vi "Weather Station UI.vi"(7 "stop":bool, 9 "Limite inférieure":dbl=10.0 min=0.0 max=50.0, 10 "Limite supérieure":dbl=30.0 min=0.0 max=50.0) -> (1 "Mise en garde":string, 2 "Historique de la température":dbl(graph))   [LabVIEW 2009]
doc: "Ceci est le VI principal du Projet Station météo. Il comporte l'interface utilisateur d'un système de mise en garde concernant la température. La température est mesurée toutes les demi-secondes ; les données sont enregistrées lorsqu'une mise en garde survient.\n\nEntrées utilisateur : Limite supérieure de température, Limite inférieure de température, Unités de température.\nSorties : Température actuelle, État de mise en garde."
uses:
  Supporting Files/Weather Station States.ctl
panel:
  in  "Limite supérieure du vent":dbl(slide)=50.0 scale=0.0..100.0
  out "Historique de la vitesse du vent":dbl(graph)
  in  "Données météo":dynamicdata(graph)
  # "Celsius"
  # "Gamme de température (C)"
  # "Canicule"
  # "Gel"
  # "km/h"
  # "Vitesse maximale du vent sans danger (km/h)"
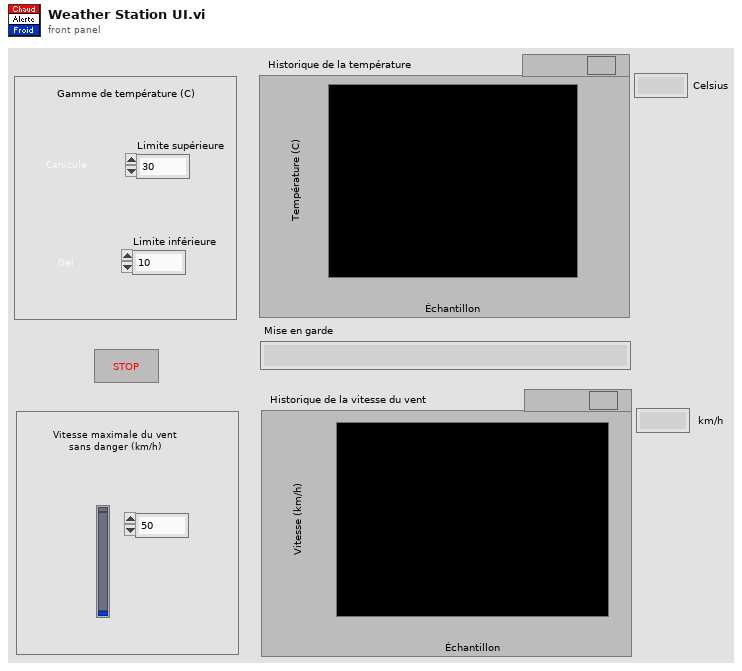
[diagram p1: front panel]
types:
  T1 = cluster{"Température":dbl, "Limite supérieure de T":dbl, "Limite inférieure de T":dbl, "Vitesse du vent":dbl, "Limite supérieure du vent":dbl, "Mise en garde":string, "Temps":dbl}
  T2 = typedef "Weather Station States.ctl" = enum16{"Analyse", "Traiter l'IU", "Définir  la mise en garde", "Enregistrement des  données", "Arrêter"}
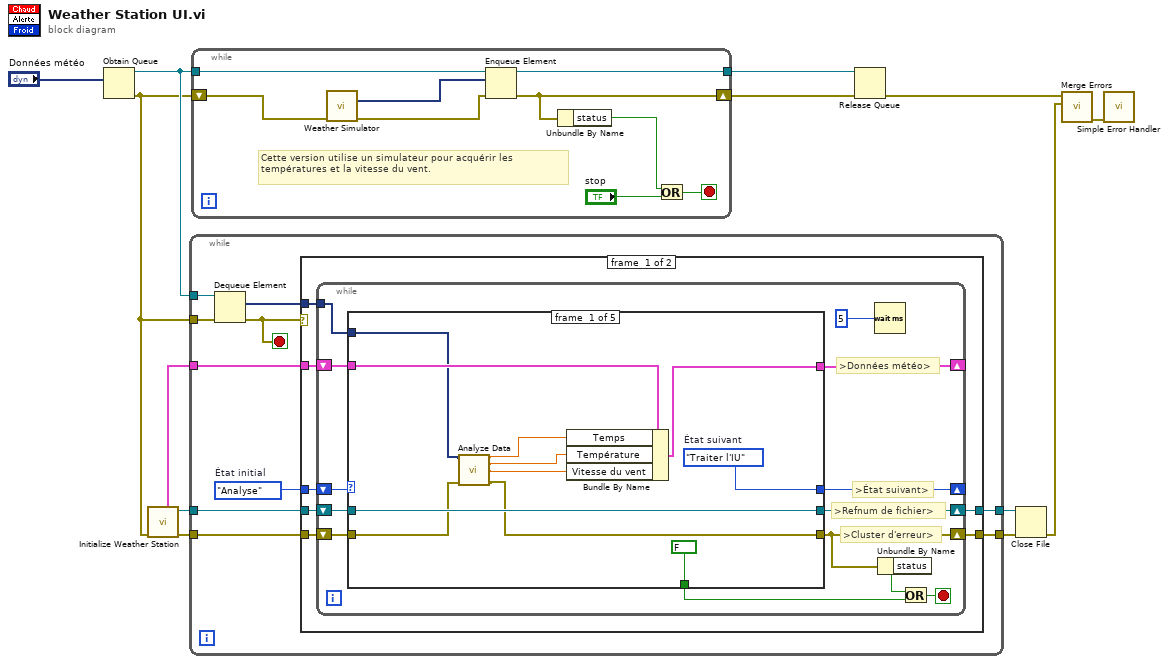
[diagram p0: block diagram]
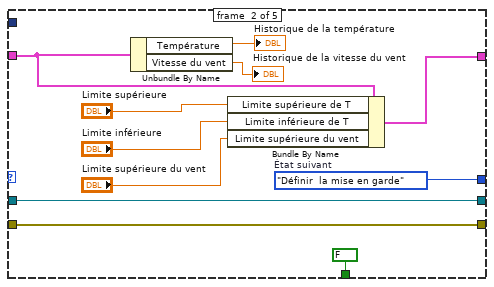
[diagram p2: hidden frame]
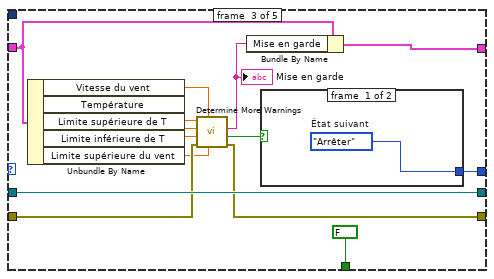
[diagram p3: hidden frame]
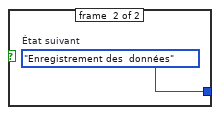
[diagram p4: hidden frame]
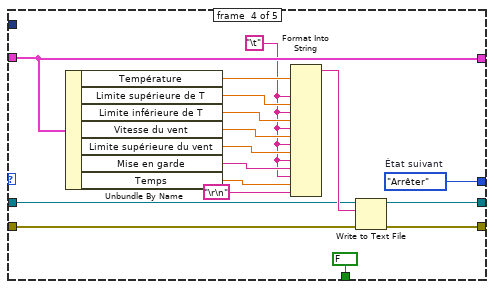
[diagram p5: hidden frame]
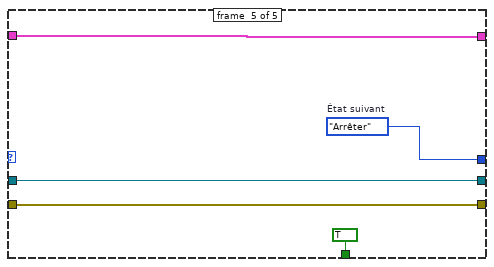
[diagram p6: hidden frame]
diagram:
  n1 = Obtain Queue ("Obtenir une file d'attente")(element data type="Données météo") -> (queue out=w5:refnum<queue>, error out=w1:errorcluster)  [unwired: 4 in, 1 out]
  n2 = call "Initialize Weather Station.vi"("entrée d'erreur (pas d'erreur)"=w1) -> ("sortie d'erreur"=w10:errorcluster, "refnum de fichier"=w11:refnum<file>, "Données météo"=w9:T1)  [unwired: 8 in]
  n3 = while "Boucle While" {
    tunnel: [w23] -> w13
    tunnel: [w22] -> w12
    tunnel: w11 -> [w21]
    tunnel: w10 -> [w20]
    tunnel: w9 -> [w19]
    tunnel: w5 -> [w18]
    tunnel: w1 -> [w17]
    stop <- w16 stop-if-true
    w14 = Weather_Station_States."Analyse"  # État initial
    n4 = Dequeue Element ("Supprimer le premier élément d'une file d'attente")(queue=w18, error in (no error)=w17) -> (element=w15:dynamicdata, error out=w16:errorcluster)  [unwired: 1 in, 2 out]
    n5 = case "Structure Condition" shown="Pas d'erreur" w16 {
      tunnel: w14 -> [w30 _]
      tunnel: [w29 w104] -> w23
      tunnel: [w28 w105] -> w22
      tunnel: w21 -> [w27 w105]
      tunnel: w20 -> [w26 w104]
      tunnel: w19 -> [w25 _]
      tunnel: w15 -> [w24 _]
      frame #0 {
        n6 = while {
          shift-right: [w42] -> _
          shift-left: w30 -> [w43]
          shift-right: [w39] -> w29
          shift-left: w26 -> [w41]
          shift-right: [w32] -> _
          shift-left: w25 -> [w36]
          shift-right: [w37] -> w28
          shift-left: w27 -> [w35]
          tunnel: w24 -> [w31]
          stop <- w40 stop-if-true
          # ">Cluster d'erreur>"
          # ">Données météo>"
          # ">Refnum de fichier>"
          # ">État suivant>"
          n7 = case shown="\"Analyse\"" w43 {
            tunnel: [w54 w59 w77 w98 w99] -> w42
            tunnel: [w47 w60 w70 w96 w101] -> w39
            tunnel: w41 -> [w48 w60 w71 w97 w101]
            tunnel: [w53 w61 w79 w95 w102] -> w37
            tunnel: [w50 w63 w72 w87 w103] -> w32
            tunnel: w36 -> [w51 w55 w73 w87 w103]
            tunnel: w35 -> [w53 w61 w79 w93 w102]
            tunnel: [FALSE ("stop") FALSE ("stop") FALSE ("stop") FALSE ("stop") TRUE ("stop")] -> w34
            tunnel: w31 -> [w49 _ _ _ _]
            frame #0 {
              w54 = Weather_Station_States."Traiter l'IU"  # État suivant
              n8 = call "Analyze Data.vi"("Données météo"=w49, "entrée d'erreur"=w48) -> ("Temps"=w44:dbl, "Température"=w45:dbl, "Vitesse du vent"=w46:dbl, "sortie d'erreur"=w47:errorcluster)  [unwired: 10 in]
              n9 = Bundle By Name(cluster=w51, "Temps"=w44, "Température"=w45, "Vitesse du vent"=w46) -> (w50:T1)
            }
            frame #1 {
              w59 = Weather_Station_States."Définir  la mise en garde"  # État suivant
              n10 = Unbundle By Name(w55) -> ("Température"=→"Historique de la température":dbl, "Vitesse du vent"=→"Historique de la vitesse du vent":dbl)
              n11 = Bundle By Name(cluster=w55, "Limite supérieure de T"="Limite supérieure", "Limite inférieure de T"="Limite inférieure", "Limite supérieure du vent"="Limite supérieure du vent") -> (w63:T1)
            }
            frame #2 {
              n12 = Unbundle By Name(w73) -> ("Vitesse du vent"=w69:dbl, "Température"=w76:dbl, "Limite supérieure de T"=w75:dbl, "Limite inférieure de T"=w74:dbl, "Limite supérieure du vent"=w68:dbl)
              n13 = call "Determine More Warnings.vi"("Vitesse max. du vent"=w68, "Vitesse actuelle du vent"=w69, "entrée d'erreur (pas d'erreur)"=w71, "Temp. min."=w74, "Temp. max."=w75, "Temp. actuelle"=w76) -> ("sortie d'erreur"=w70:errorcluster, "Mise en garde ?"=w67:bool, "Texte de mise en garde"=w66:string)  [unwired: 3 in]
              "Mise en garde" <- w66
              n14 = Bundle By Name(cluster=w73, "Mise en garde"=w66) -> (w72:T1)
              n15 = case shown="Vrai" w67 {
                tunnel: [w80 w81] -> w77
                frame #0 {
                  w80 = Weather_Station_States."Arrêter"  # État suivant
                }
                frame #1 {
                  w81 = Weather_Station_States."Enregistrement des  données"  # État suivant
                }
              }
            }
            frame #3 {
              w98 = Weather_Station_States."Arrêter"  # État suivant
              w84 = "\t" ("Tab Constant")
              n16 = Unbundle By Name(w87) -> ("Température"=w91:dbl, "Limite supérieure de T"=w90:dbl, "Limite inférieure de T"=w89:dbl, "Vitesse du vent"=w88:dbl, "Limite supérieure du vent"=w86:dbl, "Mise en garde"=w85:string, "Temps"=w83:dbl)
              n17 = Format Into String(w91, w84, w90, w84, w89, w84, w88, w84, w86, w84, w85, w84, w83, "\r\n" ("End of Line Constant")) -> (resulting string=w94:string)  [unwired: 3 in, 1 out]
              n18 = Write to Text File(file (use dialog)=w93, text=w94, error in=w97) -> (refnum out=w95:refnum<file>, error out=w96:errorcluster)  [unwired: 1 in, 1 out]
            }
            frame #4 {
              w99 = Weather_Station_States."Arrêter"  # État suivant
            }
          }
          n19 = Wait (ms)(milliseconds to wait=u32 5 ("y")) -> ()  [unwired: 1 out]
          n20 = Unbundle By Name(w39) -> ("status"=w38:bool)
          n21 = Or(x=w38, y=w34) -> (x .or. y?=w40:bool)
        }
      }
      frame #1 {
      }
    }
  }
  n22 = while "Boucle While" {
    tunnel: w5 -> [w114]
    tunnel: [w113] -> w7
    shift-right: [w110] -> w6
    shift-left: w1 -> [w106]
    stop <- w112 stop-if-true
    # "Cette version utilise un simulateur pour acquérir les températures et la vitesse du vent."
    n23 = call "Weather Simulator.vi"("entrée d'erreur (pas d'erreur)"=w106) -> ("Graphe"=w107:dynamicdata, "sortie d'erreur"=w108:errorcluster)  [unwired: 13 in]
    n24 = Enqueue Element ("Ajouter un élément à la fin d'une file d'attente")(queue=w114, element=w107, error in (no error)=w108) -> (queue out=w113:refnum<queue>, error out=w110:errorcluster)  [unwired: 1 in, 1 out]
    n25 = Unbundle By Name ("Désassembler par nom")(w110) -> ("status"=w109:bool)
    n26 = Or ("OU")(x=w109, y="stop") -> (x .or. y?=w112:bool)
  }
  n27 = Release Queue ("Libérer une file d'attente")(queue=w7, error in (no error)=w6) -> (error out=w4:errorcluster)  [unwired: 1 in, 2 out]
  n28 = Close File ("Fermer un fichier")(refnum=w12, error in=w13) -> (error out=w3:errorcluster)  [unwired: 1 out]
  n29 = call <vilib>:"Merge Errors.vi"("error in 2 (no error)"=w3, "error in 1 (no error)"=w4) -> ("error out"=w2:errorcluster)  [unwired: 5 in]
  n30 = call <vilib>:"Simple Error Handler.vi"("error in (no error)"=w2) -> ()  [unwired: 4 in, 5 out]
